vi "Termometro.vi"() -> ()   [LabVIEW 2021]
panel:
  out "Temperatura °F":dbl
  out "Peligro":bool
  out "Precaucion":bool
  out "Normal":bool
  in  "Dial":dbl(knob) scale=0.0..100.0
  out "Thermometer":dbl(slide) scale=0.0..100.0
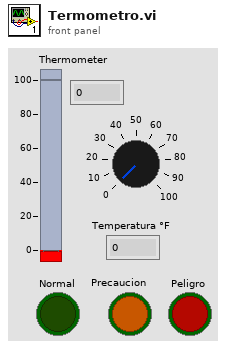
[diagram p1: front panel]
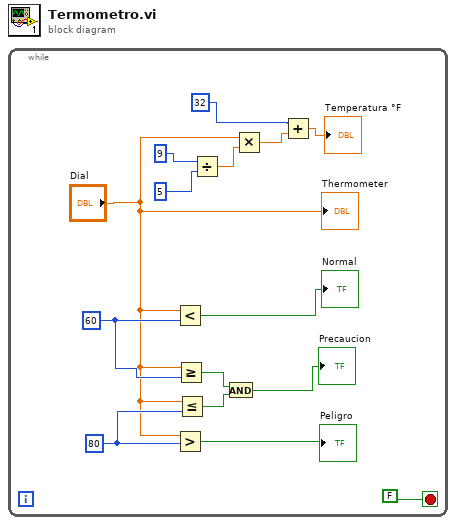
[diagram p0: block diagram]
diagram:
  n1 = while {
    stop <- FALSE stop-if-true
    w12 = 80
    w11 = 60
    n2 = Less?(x="Dial", y=w11) -> (x < y?=→"Normal":bool)
    n3 = Greater?(x="Dial", y=w12) -> (0:→"Peligro":bool)
    n4 = Greater Or Equal?(x="Dial", y=w11) -> (x >= y?=w9:bool)
    n5 = Less Or Equal?(x="Dial", y=w12) -> (x <= y?=w8:bool)
    n6 = Divide(x=9, y=5) -> (x/y=w13:dbl)
    n7 = And(x=w9, y=w8) -> (x .and. y?=→"Precaucion":bool)
    n8 = Multiply(x="Dial", y=w13) -> (x*y=w3:dbl)
    n9 = Add(x=32, y=w3) -> (x+y=→"Temperatura °F":dbl)
    "Thermometer" <- "Dial"
  }
